vi "Test.vi"() -> ()   [LabVIEW 2024]
uses:
  Message/Message.lvclass
  PID Loop/PID Loop/PID Loop.lvclass
  PID Loop/PID/PID.lvclass
  C:/Users/uspoaotto/OneDrive - Oregon Tool/Desktop/working copies/helperLoop/src/OOQMH/Message/Message.lvclass
  Stop/Stop.lvclass
  Start Polling/Start Polling.lvclass
  Set Polling Message/Set Polling Message.lvclass
  Stop Polling/Stop Polling.lvclass
  PID Loop/Set Loop Period/Set Loop Period.lvclass
panel:
  in  "Loop Period in ms":u32=10
  in  "Stop":bool
  in  "Stop Polling":bool
  in  "Start Polling":bool
  in  "Launch PID Loop":bool
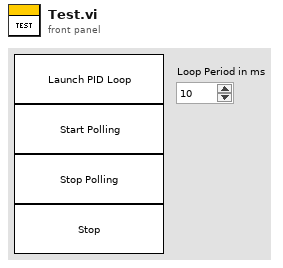
[diagram p1: front panel]
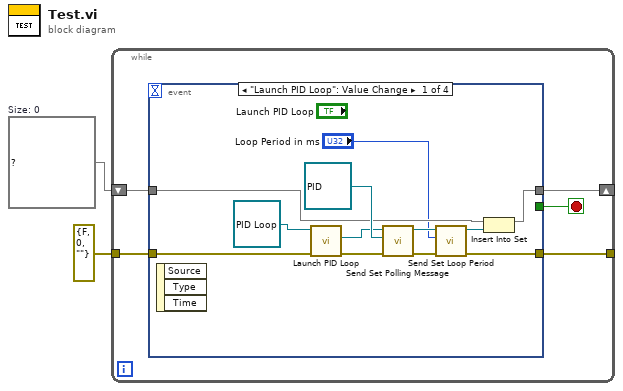
[diagram p0: block diagram]
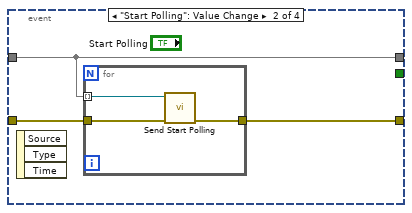
[diagram p2: hidden frame]
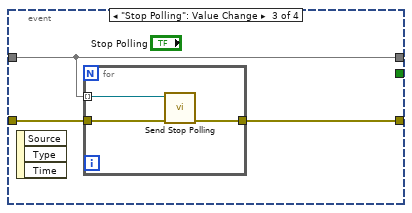
[diagram p3: hidden frame]
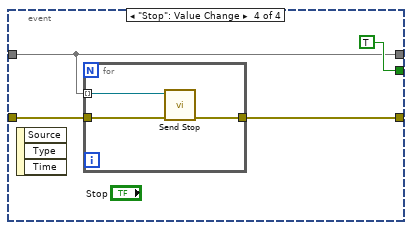
[diagram p4: hidden frame]
diagram:
  w2 = set{refnum<queue>} {}  # Size: 0
  n1 = while {
    shift-right: [w5] -> _
    shift-left: w2 -> [w6]
    tunnel: [w4] -> _
    tunnel: errorcluster {"status"=FALSE, "code"=0, "source"=""} ("error constant") -> [w3]
    stop <- w7 stop-if-true
    n2 = event shown="[0] \"Launch PID Loop\": Value Change" {
      selector: _ -> [_ _ _ _]
      dyn-events: _ -> [_ _ _ _]
      timeout: _ -> [_ _ _ _]
      tunnel: [_ _ _ TRUE] -> w7
      tunnel: w6 -> [w16 w22 w28 w34]
      tunnel: [w15 w22 w28 w34] -> w5
      tunnel: [w9 w20 w26 w32] -> w4
      tunnel: w3 -> [w13 w21 w27 w33]
      event "Launch PID Loop": Value Change {
        n3 = event-data() -> ()  [unwired: 1 in, 3 out]
        n4 = call "Launch PID Loop.vi"("error in (no error)"=w13, "PID Loop in"=refnum<class "PID Loop.lvclass"> refnum ("PID Loop.lvlib:PID Loop.lvclass")) -> ("error out"=w14:errorcluster, "Message Queue"=w17:refnum<queue>)  [unwired: 8 in]
        n5 = call "Send Set Polling Message.vi"("error in (no error)"=w14, "Polling Message"=refnum<class "PID.lvclass"> refnum ("PID Loop.lvlib:PID.lvclass"), "Message Queue in"=w17) -> ("error out"=w10:errorcluster, "Message Queue out"=w12:refnum<queue>)  [unwired: 7 in]
        n6 = call "Send Set Loop Period.vi"("error in (no error)"=w10, "Loop Period in ms (10)"="Loop Period in ms", "Message Queue in"=w12) -> ("error out"=w9:errorcluster, "Message Queue out"=w11:refnum<queue>)  [unwired: 7 in]
        n7 = Insert Into Set(10:w11, 11:w16) -> (3:w15:set{refnum<queue>})  [unwired: 1 out]
      }
      event "Start Polling": Value Change {
        n8 = event-data() -> ()  [unwired: 1 in, 3 out]
        n9 = for {
          tunnel: w22 -> [w25] mode=indexing
          tunnel: w21 -> [w24]
          tunnel: [w23] -> w20
          n10 = call "Send Start Polling.vi"("error in (no error)"=w24, "Message Queue in"=w25) -> ("error out"=w23:errorcluster)  [unwired: 8 in, 1 out]
        }
      }
      event "Stop Polling": Value Change {
        n11 = event-data() -> ()  [unwired: 1 in, 3 out]
        n12 = for {
          tunnel: w28 -> [w31] mode=indexing
          tunnel: w27 -> [w30]
          tunnel: [w29] -> w26
          n13 = call "Send Stop Polling.vi"("error in (no error)"=w30, "Message Queue in"=w31) -> ("error out"=w29:errorcluster)  [unwired: 8 in, 1 out]
        }
      }
      event "Stop": Value Change {
        n14 = event-data() -> ()  [unwired: 1 in, 3 out]
        n15 = for {
          tunnel: w34 -> [w38] mode=indexing
          tunnel: w33 -> [w37]
          tunnel: [w36] -> w32
          n16 = call "Send Stop.vi"("error in (no error)"=w37, "Message Queue in"=w38) -> ("error out"=w36:errorcluster)  [unwired: 9 in]
        }
      }
    }
  }
